vi "PCO_SetActiveLookupTable.vi"(8 "error in (no error)":errorcluster {"code" format="%x"}, 9 "wOffset":u16, 10 "wIdentifier":u16, 11 "ph":u64) -> (0 "error out":errorcluster {"code" format="%x"}, 2 "ErrorMessage":i32 format="%x", 3 "ph out":u64)   [LabVIEW 2020, in "SDK.lvlib" / "ImageSensor.lvlib"]
doc: "<b>Description:</b>\nThis function does set an active lookup table (LUT) in the camera. If wIdentifier is set to 0 while calling this function, the lookup table functionality will be disabled and data values from the sensor are directly send to the interface. If wIdentifier is one of the available LUT identifiers of the camera data handling is as follows: at first the offset value given by parameter wOffset is subtracted from the data values from the sensor. The resulting value is the input to the current selected LUT.\nValid values for the LUT identifier wIdentifier can be retrieved with function PCO_GetLookuptableInfo.\n\n<b>Supported camera type:</b>\npco.edge\n\n<b>Descriptor dependency:</b>\nNone"
uses:
  ImageSensor.lvlib
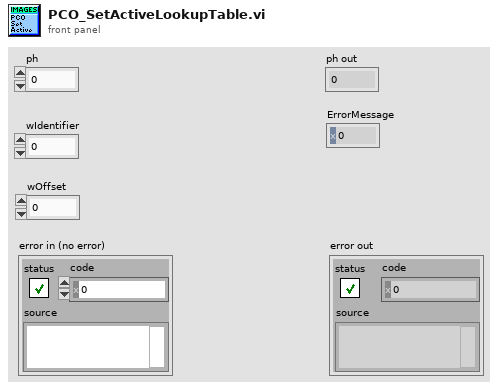
[diagram p1: front panel]
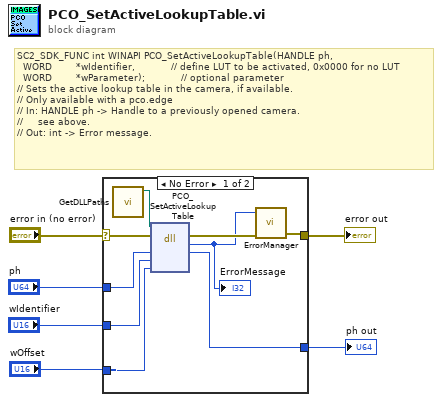
[diagram p0: block diagram]
diagram:
  # "SC2_SDK_FUNC int WINAPI PCO_SetActiveLookupTable(HANDLE ph,\n  WORD        *wIdentifier,            // define LUT to be activated, 0x0000 for no LUT\n  WORD        *wParameter);            // optional parameter\n// Sets the active lookup table in the camera, if available.\n// Only available with a pco.edge\n// In: HANDLE ph -> Handle to a previously opened camera.\n//     see above.\n// Out: int -> Error message."
  n1 = case shown="No Error" "error in (no error)" {
    selector: "error in (no error)" -> [w11 w17]
    tunnel: "ph" -> [w15 w16]
    tunnel: [w14 w16] -> w5
    tunnel: [w9 w17] -> w4
    tunnel: "wIdentifier" -> [w13 _]
    tunnel: "wOffset" -> [w12 _]
    frame No Error {
      n2 = call "GetDLLPaths.vi"() -> ("SC2_Cam_Path"=w7:path)  [unwired: 9 in, 2 out]
      n3 = dll-call lib="?" fn="PCO_SetActiveLookupTable"(path in=w7, error in=w11, "ph"=w15, "wIdentifier"=w13, "wOffset"=w12) -> (error out=w10:errorcluster, "return type"=w8:i32, "ph"=w14:u64)  [unwired: 3 in, 1 out]
      "ErrorMessage" <- w8
      n4 = call "ErrorManager.vi"("error in (no error)"=w10, "error code"=w8) -> ("error out"=w9:errorcluster)  [unwired: 3 in]
    }
    frame Error {
    }
  }
  "ph out" <- w5
  "error out" <- w4
